vi "Get SMO RC Type.vi"(8 "error in (no error)":errorcluster, 11 "ExampleInstrument in":refnum<class "LevyLab Instrument.lvclass">) -> (0 "error out":errorcluster, 2 "Configuration.SMO.RC Type":T1=enum."STM", 3 "ExampleInstrument out":refnum<class "LevyLab Instrument.lvclass">)   [LabVIEW 2020, in "LevyLab Instrument.lvclass"]
uses:
  LevyLab Instrument.lvclass
  SMOs/Instrument/Typedefs/SMO RC Type--enum.ctl
  SMOs/Instrument/Instrument.lvclass
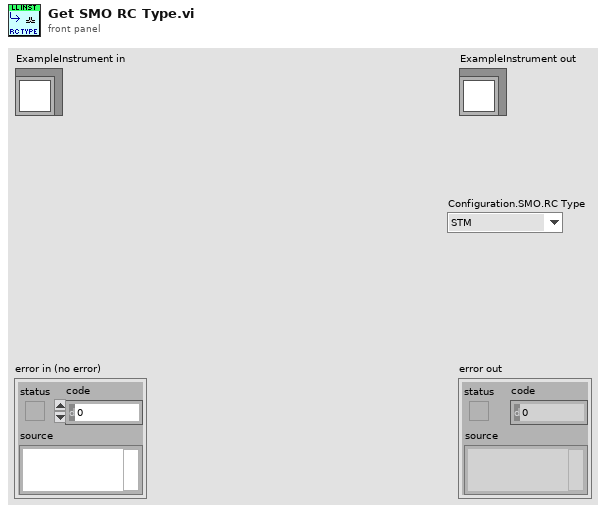
[diagram p1: front panel]
types:
  T1 = typedef "Instrument.lvclass/SMO RC Type--enum.ctl" = enum16{"RC", "STM", "ZMQ"}
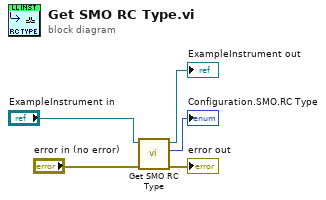
[diagram p0: block diagram]
diagram:
  n1 = call-parent "Get SMO RC Type.vi"("error in (no error)"="error in (no error)", "Instrument in"="ExampleInstrument in") -> ("error out"=→"error out":errorcluster, "Configuration.SMO.RC Type"=→"Configuration.SMO.RC Type":T1, "Instrument out"=→"ExampleInstrument out":refnum<class "LevyLab Instrument.lvclass">)  [unwired: 7 in]
